vi "CAlculateingAverageTemp.vi"() -> ()   [LabVIEW 2024]
panel:
  out "Waveform Chart 2":dbl(graph)
  in  "Stop Button":bool
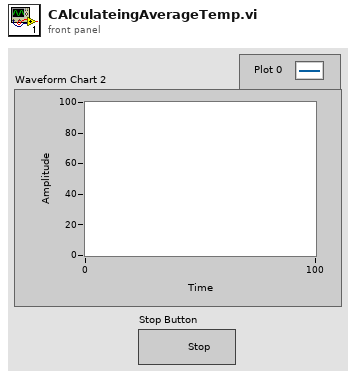
[diagram p1: front panel]
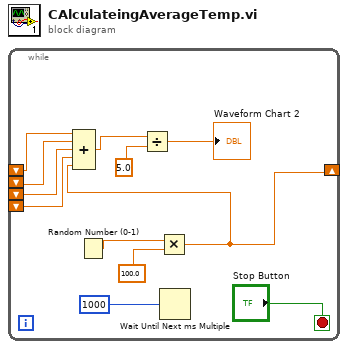
[diagram p0: block diagram]
diagram:
  n1 = while {
    shift-right: [w5] -> _
    shift-left: _ -> [w9]
    shift-left: _ -> [w8]
    shift-left: _ -> [w7]
    shift-left: _ -> [w6]
    stop <- "Stop Button" stop-if-true
    n2 = Random Number (0-1)() -> (number: 0 to 1=w11:dbl)
    n3 = Multiply(x=w11, y=100.0) -> (x*y=w5:dbl)
    n4 = Compound Arithmetic op=ADD(w9, w8, w7, w6, w5) -> (w4:dbl)
    n5 = Divide(x=w4, y=5.0) -> (x/y=→"Waveform Chart 2":dbl)
    n6 = Wait Until Next ms Multiple(millisecond multiple=u32 1000) -> ()  [unwired: 1 out]
  }
